vi "Check Cust Device Connected Status.vi"(2 "WkspRef":T2, 3 "Link":T1) -> (0 "connected?":bool)   [LabVIEW 2011]
uses:
  <vilib>/NI Veristand/Execution/Workspace/WorkspaceAPI.ctl
  NationalInstruments.VeriStand.ClientAPI
  Controls/ECUMC Item.ctl
  <vilib>/NI Veristand/Execution/Workspace/NI VeriStand - Get Multiple Channel Values.vi
  <vilib>/NI Veristand/Execution/Workspace/NI_VS Workspace ExecutionAPI.lvlib
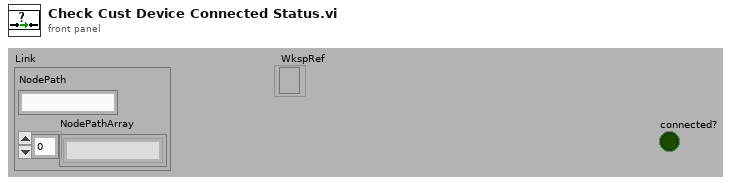
[diagram p1: front panel]
types:
  T1 = typedef "ECUMC Item.ctl" = cluster{"NodePath":string, "NodePathArray":string[]}
  T2 = typedef "NI_VS Workspace ExecutionAPI.lvlib/WorkspaceAPI.ctl" = refnum<k24>
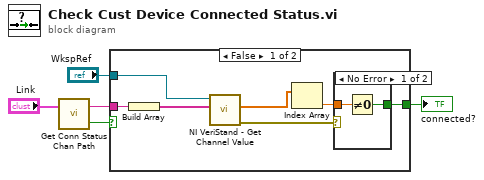
[diagram p0: block diagram]
diagram:
  n1 = call "Get Conn Status Chan Path.vi"("Link"="Link") -> ("Empty Link?"=w3:bool, "Conn Status Chan"=w4:string)  [unwired: 1 in]
  n2 = case shown="False" w3 {
    tunnel: [w12 _] -> w5
    tunnel: w4 -> [w11 _]
    tunnel: "WkspRef" -> [w8 _]
    frame False {
      n3 = Build Array(w11) -> (w7:string[])
      n4 = call-poly <vilib>:"NI VeriStand - Get Channel Value.vi"("Channels"=w7, "WorkspaceManager in"=w8) -> ("error out"=w9:errorcluster, "Values"=w10:dbl[])  [unwired: 7 in, 1 out]
      n5 = Index Array(array=w10) -> (element=w6:dbl)  [unwired: 1 in]
      n6 = case shown="No Error" w9 {
        tunnel: w6 -> [w14 _]
        tunnel: [w13 _] -> w12
        frame No Error {
          n7 = Not Equal To 0?(x=w14) -> (x != 0?=w13:bool)
        }
        frame Error {
        }
      }
    }
    frame True {
    }
  }
  "connected?" <- w5
